vi "Complete Collection.vi"(8 "error in":errorcluster) -> (0 "error out":errorcluster)   [LabVIEW 2013]
uses:
  Collection Support/Controls/PED States.ctl
  Collection Support/Controls/FirstCall.ctl
panel:
  in  "Trial Duration (s)":dbl=10.0 format="%#_13g"
  in  "Exit Button":bool
  in  "Longest Time Between Interruptions":dbl=1.3 format="%#_13g"
  in  "Starting Second":dbl=3.4 format="%#_13g"
  in  "Interruptions":i32
  in  "Delay":u32
  in  "Shortest Time Between Interruptions":dbl=0.8 format="%#_13g"
  out "Countdown":dbl format="%#.0g"
  out "Audio Chart":dynamicdata(graph)
  out "Pressure Chart":dynamicdata(graph)
  in  "START/STOP":bool
  in  "Stopped?":bool
  out "STOP":bool
  out "GO":bool
  # "- You can set the delay and number of interruptions to 0 to test labial interruptions\n\n-The starting second sets how long after GO the first interruption will be\n\n-The longest time between interrruptions sets the maximum amount of time between interruptions\n\n-The shortest time between interruptions sets the minimum time between interruptions. If you want quicker intteruptions, lower this value."
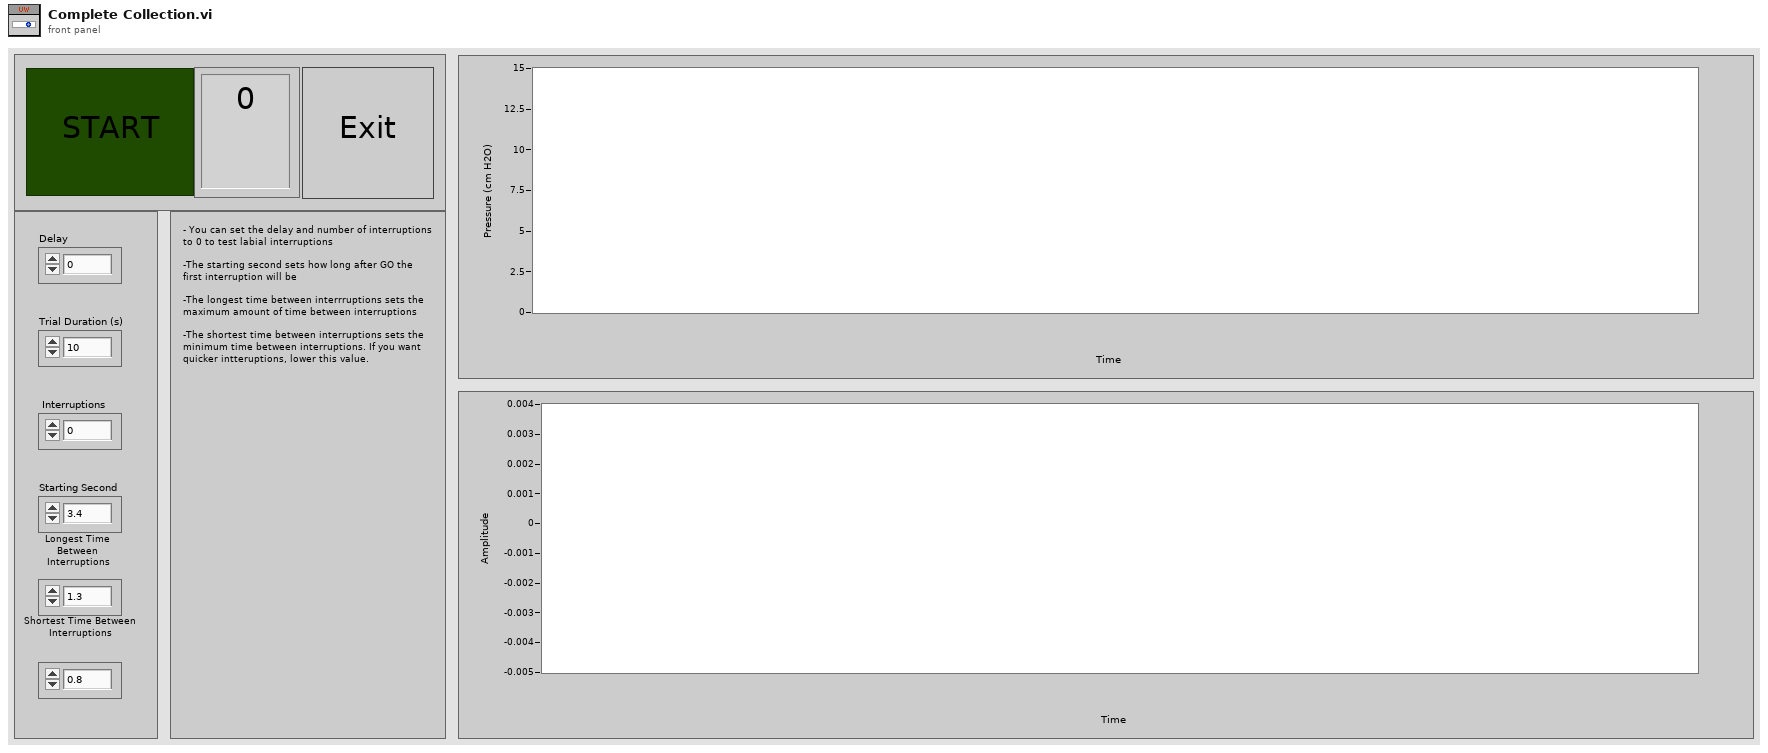
[diagram p1: front panel]
types:
  T1 = enum16{"open", "replace", "create", "open or create", "replace or create", "replace or create with confirmation"}
  T2 = typedef "PED States.ctl" = enum16{"Initialize", "Wait", "Record", "Save", "Reset", "Exit"}
  T3 = typedef "FirstCall.ctl" = enum16{"First", "After"}
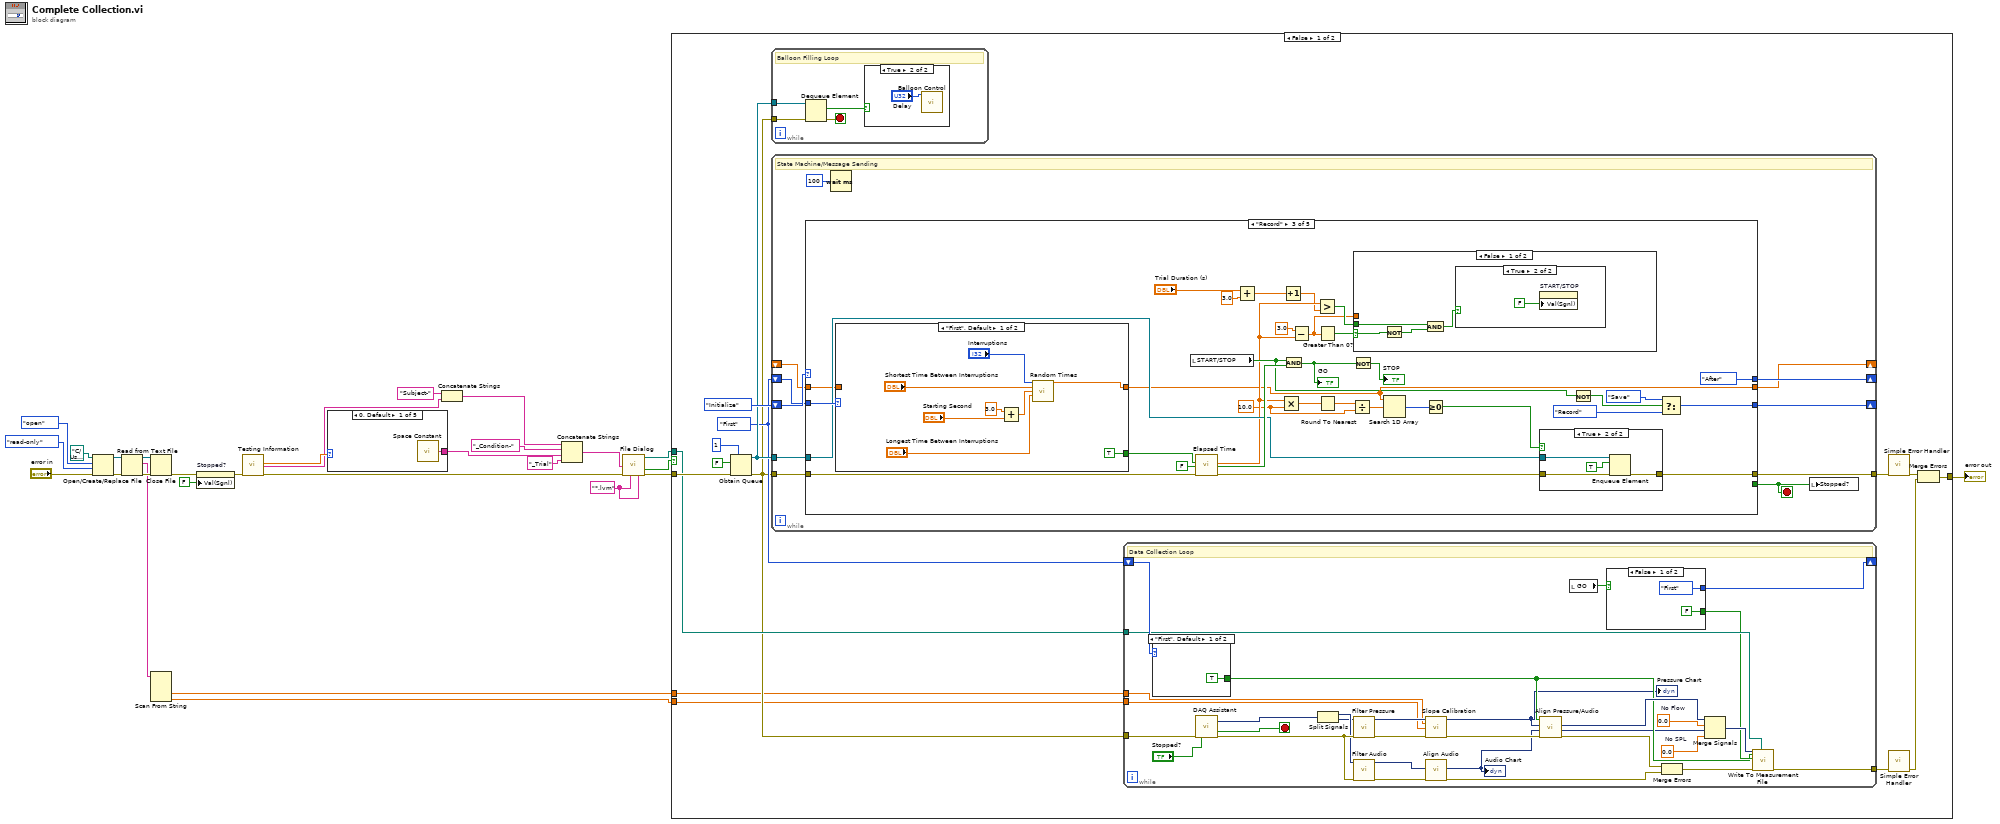
[diagram p0: block diagram]
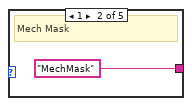
[diagram p2: hidden frame]
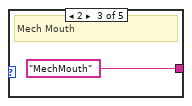
[diagram p3: hidden frame]
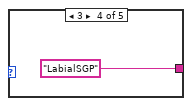
[diagram p4: hidden frame]
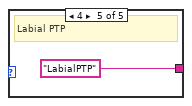
[diagram p5: hidden frame]
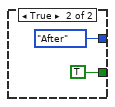
[diagram p6: hidden frame]
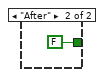
[diagram p7: hidden frame]
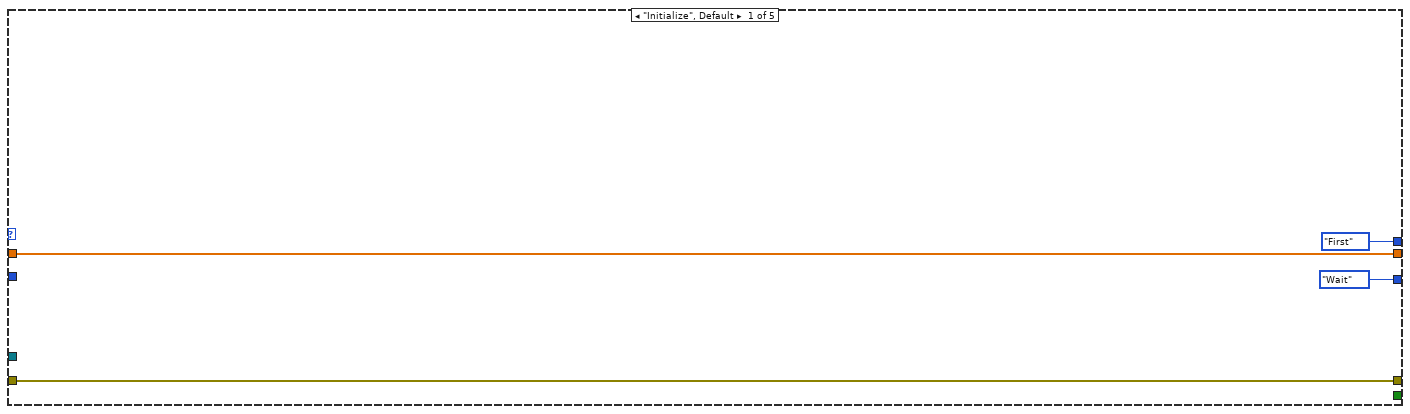
[diagram p9: hidden frame]
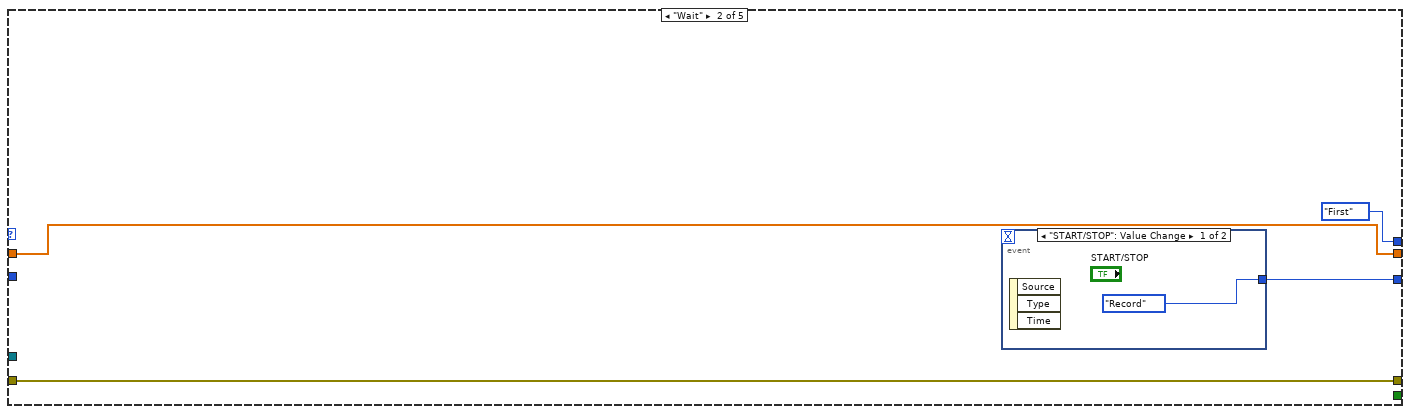
[diagram p10: hidden frame]
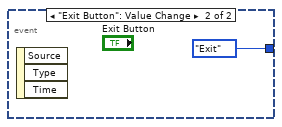
[diagram p11: hidden frame]
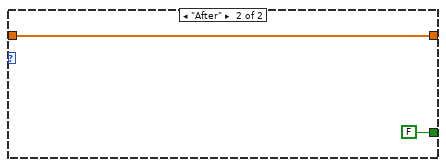
[diagram p13: hidden frame]
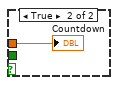
[diagram p15: hidden frame]
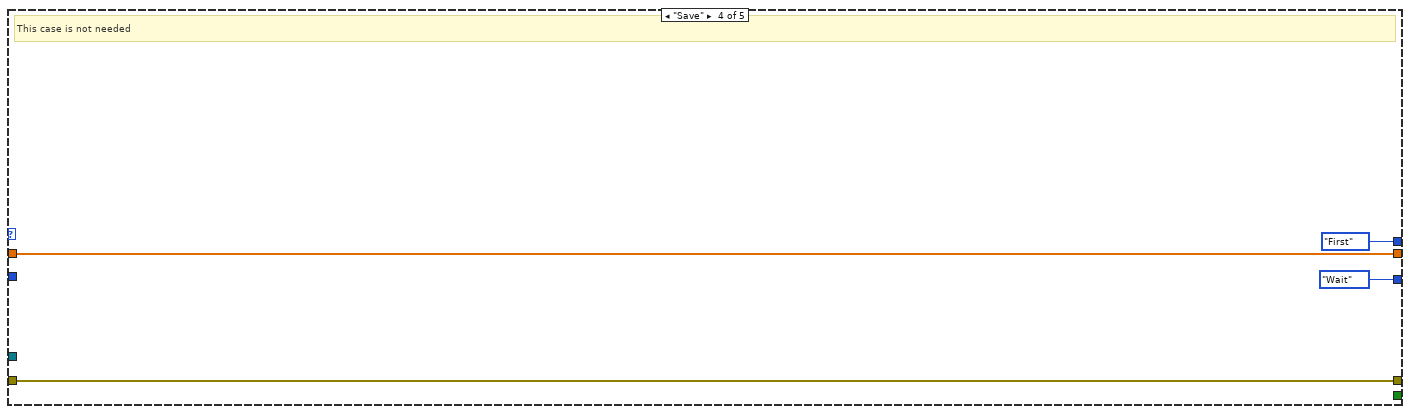
[diagram p16: hidden frame]
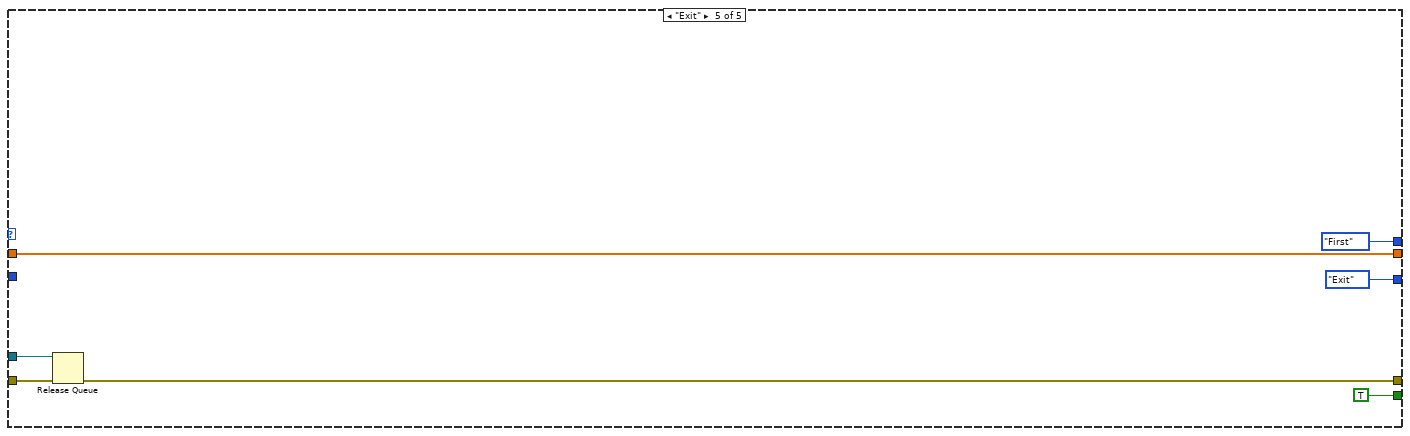
[diagram p17: hidden frame]
diagram:
  w26 = "*.lvm" ("pattern label")
  n1 = Open/Create/Replace File(file path (use dialog)=path "C:/Users/scholp/Desktop/Calibration .txt files/Calibration Values.txt", error in="error in", operation (0:open)=T1."open", access (0:read/write)=enum16{"read/write", "read-only", "write-only"}."read-only") -> (refnum out=w20:refnum<file>, error out=w24:errorcluster)  [unwired: 2 in, 1 out]
  n2 = Read from Text File(file (use dialog)=w20, error in=w24) -> (refnum out=w18:refnum<file>, text=w17:string, error out=w23:errorcluster)  [unwired: 2 in, 1 out]
  n3 = Close File(refnum=w18, error in=w23) -> (error out=w14:errorcluster)  [unwired: 1 out]
  n4 = Scan From String(input string=w17) -> (output 1=w16:dbl, output 2=w15:dbl)  [unwired: 5 in, 3 out]
  n5 = property on="Stopped?" class="Bool (strict)"(error in=w14, "Val(Sgnl)"=FALSE ("Value (Signaling)")) -> (error out=w1:errorcluster)  [unwired: 1 in, 1 out]
  n6 = call "Testing Information"("error in (no error)"=w1) -> ("Condition"=w10:dbl, "Subject"=w8:string, "error out"=w2:errorcluster)  [unwired: 15 in, 1 out]
  n7 = case shown="0, Default" w10 {
    tunnel: [w29 "MechMask" ("string") "MechMouth" ("string") "LabialSGP" ("string") "LabialPTP" ("string")] -> w7
    frame 0, Default {
      n8 = call <vilib>:"Space Constant.vi"() -> ("String"=w29:string)
    }
    frame 1 {
      # "Mech Mask"
    }
    frame 2 {
      # "Mech Mouth"
    }
    frame 3 {
    }
    frame 4 {
      # "Labial PTP"
    }
  }
  n9 = Concatenate Strings("Subject-" ("default name"), w8) -> (w4:string)
  n10 = Concatenate Strings(w4, "_Condition-" ("string"), w7, "_Trial" ("string")) -> (w3:string)
  n11 = call "File Dialog"("default name"=w3, "error in"=w2, "pattern (all files)"=w26, "pattern label"=w26) -> ("selected path"=w27:path, "cancelled"=w12:bool, "error out"=w28:errorcluster)  [unwired: 8 in, 1 out]
  n12 = case shown="False" w12 {
    tunnel: w28 -> [w43 w177]
    tunnel: w27 -> [w42 _]
    tunnel: w16 -> [w38 _]
    tunnel: w15 -> [w37 _]
    tunnel: [w34 w177] -> w11
    frame False {
      w44 = FirstCall."First"
      n13 = Obtain Queue(max queue size (-1, unlimited)=1, element data type=FALSE, error in (no error)=w43) -> (queue out=w45:refnum<queue>, error out=w41:errorcluster)  [unwired: 2 in, 1 out]
      n14 = while {
        tunnel: w45 -> [w87]
        tunnel: w41 -> [w86]
        stop <- w88 stop-if-true
        # "Balloon Filling Loop"
        n15 = Dequeue Element(queue=w87, error in (no error)=w86) -> (element=w89:bool, error out=w88:errorcluster)  [unwired: 1 in, 2 out]
        n16 = case shown="True" w89 {
          frame False {
          }
          frame True {
            n17 = call "Balloon Control.vi"("Delay (ms)"="Delay") -> ()  [unwired: 11 in]
          }
        }
      }
      n18 = while {
        shift-right: [w101] -> _
        shift-left: PED_States."Initialize" -> [w100]
        tunnel: w45 -> [w97]
        tunnel: w41 -> [w99]
        shift-right: [w96] -> _
        shift-left: w44 -> [w98]
        tunnel: [w94] -> w39
        shift-right: [w91] -> _
        shift-left: _ -> [w92]
        stop <- w95 stop-if-true
        # "State Machine/Message Sending"
        n19 = case shown="\"Record\"" w100 {
          tunnel: [_ _ _ _ TRUE] -> w95
          tunnel: [PED_States."Wait" ("f") w109 w128 PED_States."Wait" ("element") PED_States."Exit" ("element")] -> w101
          tunnel: w99 -> [w103 w106 w134 w167 w174]
          tunnel: w98 -> [_ _ w130 _ _]
          tunnel: w97 -> [_ _ w122 _ w173]
          tunnel: [FirstCall."First" FirstCall."First" FirstCall."After" FirstCall."First" FirstCall."First"] -> w96
          tunnel: [w102 w107 w118 w166 w170] -> w91
          tunnel: [w103 w106 w121 w167 w171] -> w94
          tunnel: w92 -> [w102 w107 w117 w166 w170]
          frame "Initialize", Default {
          }
          frame "Wait" {
            n20 = event shown="[0] \"START/STOP\": Value Change" {
              selector: _ -> [_ _]
              dyn-events: _ -> [_ _]
              timeout: _ -> [_ _]
              tunnel: [PED_States."Record" ("element") PED_States."Exit" ("element")] -> w109
              event "START/STOP": Value Change {
                n21 = event-data() -> ()  [unwired: 1 in, 3 out]
              }
              event "Exit Button": Value Change {
                n22 = event-data() -> ()  [unwired: 1 in, 3 out]
              }
            }
          }
          frame "Record" {
            w112 = 10.0 ("x")
            n23 = case shown="\"First\", Default" w130 {
              tunnel: [TRUE FALSE] -> w131
              tunnel: [w156 w158] -> w118
              tunnel: w117 -> [_ w158]
              frame "First", Default {
                n24 = Add(x=3.0, y="Starting Second") -> (x+y=w150:dbl)
                n25 = call "Random Times.vi"("Number of Interruptions"="Interruptions", "Start Second"="Shortest Time Between Interruptions", "Longest Gap"=w150, "Shortest Gap"="Longest Time Between Interruptions") -> ("Interruption TImes"=w156:dbl[])  [unwired: 10 in, 1 out]
              }
              frame "After" {
              }
            }
            n26 = local read "START/STOP"() -> (w135:bool)
            n27 = call "Elapsed Time"("Reset"=w131, "Auto Reset"=FALSE, "error in (no error)"=w134) -> ("Elapsed Time (s)"=w120:dbl, "Time has Elapsed"=w138:bool, "error out"=w123:errorcluster)  [unwired: 9 in, 5 out]
            n28 = Add(x="Trial Duration (s)", y=3.0) -> (x+y=w113:dbl)
            n29 = Multiply(x=w120, y=w112) -> (x*y=w125:dbl)
            n30 = Increment(x=w113) -> (x+1=w116:dbl)
            n31 = And(x=w135, y=w138) -> (x .and. y?=w137:bool)
            "GO" <- w137
            n32 = Subtract(x=3.0, y=w120) -> (x-y=w139:dbl)
            n33 = Greater?(x=w120, y=w116) -> (0:w141:bool)
            n34 = Greater Than 0?(x=w139) -> (x > 0?=w142:bool)
            n35 = Round To Nearest(number=w125) -> (nearest integer value=w124:dbl)
            n36 = Divide(x=w124, y=w112) -> (x/y=w126:dbl)
            n37 = Not(x=w137) -> (.not. x?=→"STOP":bool)
            n38 = case shown="False" w142 {
              selector: w142 -> [w161 _]
              tunnel: w139 -> [_ w165]
              tunnel: w141 -> [w163 _]
              frame False {
                n39 = Not(x=w161) -> (.not. x?=w160:bool)
                n40 = And(x=w163, y=w160) -> (x .and. y?=w162:bool)
                n41 = case shown="True" w162 {
                  frame False {
                  }
                  frame True {
                    n42 = property on="START/STOP" class="Bool (strict)"("Val(Sgnl)"=FALSE ("Value (Signaling)")) -> ()  [unwired: 2 in, 2 out]
                  }
                }
              }
              frame True {
                "Countdown" <- w165
              }
            }
            n43 = Search 1D Array(1D array=w118, element=w126) -> (index of element=w127:i32)  [unwired: 1 in]
            n44 = Greater Or Equal To 0?(x=w127) -> (x >= 0?=w119:bool)
            n45 = case shown="True" w119 {
              tunnel: [w145 w149] -> w121
              tunnel: w123 -> [w145 w148]
              tunnel: w122 -> [_ w147]
              frame False {
              }
              frame True {
                n46 = Enqueue Element(queue=w147, element=TRUE, error in (no error)=w148) -> (error out=w149:errorcluster)  [unwired: 1 in, 2 out]
              }
            }
            n47 = Not(x=w135) -> (.not. x?=w133:bool)
            n48 = Select(t=PED_States."Save" ("f"), s=w133, f=PED_States."Record") -> (s? t:f=w128:T2)
          }
          frame "Save" {
            # "This case is not needed"
          }
          frame "Exit" {
            n49 = Release Queue(queue=w173, error in (no error)=w174) -> (error out=w171:errorcluster)  [unwired: 1 in, 2 out]
          }
        }
        n50 = Wait (ms)(milliseconds to wait=u32 100) -> ()  [unwired: 1 out]
        n51 = local write "Stopped?"(w95) -> ()
      }
      n52 = while {
        tunnel: w41 -> [w72]
        shift-right: [w66] -> _
        shift-left: w44 -> [w68]
        tunnel: w42 -> [w65]
        tunnel: [w61] -> w40
        tunnel: w38 -> [w60]
        tunnel: w37 -> [w59]
        stop <- w73 stop-if-true
        w55 = 0.0  # No SPL
        w56 = 0.0  # No Flow
        # "Data Collection Loop"
        n53 = case shown="\"First\", Default" w68 {
          tunnel: [TRUE FALSE] -> w52
          frame "First", Default {
          }
          frame "After" {
          }
        }
        n54 = call "DAQ Assistant"("error in"=w72, "stop (F)"="Stopped?") -> ("data"=w76:dynamicdata, "stopped"=w73:bool, "error out"=w58:errorcluster)  [unwired: 14 in, 1 out]
        n55 = Split Signals(w76) -> (w54:dynamicdata, w53:dynamicdata)  [unwired: 2 in]
        n56 = call "Filter Pressure"("error in (no error)"=w58, "Signal"=w53) -> ("error out"=w75:errorcluster, "Filtered Signal"=w79:dynamicdata)  [unwired: 8 in]
        n57 = call "Filter Audio"("error in (no error)"=w58, "Signal"=w54) -> ("error out"=w77:errorcluster, "Filtered Signal"=w78:dynamicdata)  [unwired: 8 in]
        n58 = call "Slope Calibration.vi"("Voltage"=w79, "Slope"=w60, "Intercept"=w59, "error in (no error)"=w75) -> ("Result"=w49:dynamicdata, "error out"=w74:errorcluster)  [unwired: 10 in]
        "Pressure Chart" <- w49
        n59 = call "Align Audio"("error in (no error)"=w77, "Signals"=w78) -> ("error out"=w69:errorcluster, "Resampled Signals"=w51:dynamicdata)  [unwired: 7 in, 1 out]
        "Audio Chart" <- w51
        n60 = call "Align Pressure/Audio"("error in (no error)"=w74, "Signals 2"=w51, "Signals"=w49, "Reset"=w52) -> ("error out"=w70:errorcluster, "Resampled Signals 2"=w50:dynamicdata, "Resampled Signals"=w57:dynamicdata)  [unwired: 5 in]
        n61 = local read "GO"() -> (w67:bool)
        n62 = case shown="False" w67 {
          tunnel: [FirstCall."First" FirstCall."After"] -> w66
          tunnel: [FALSE TRUE] -> w62
          frame False {
          }
          frame True {
          }
        }
        n63 = Merge Errors(w70, w69) -> (w63:errorcluster)
        n64 = Merge Signals(w57, w56, w50, w55) -> (w64:dynamicdata)
        n65 = call "Write To Measurement File"("Signals"=w64, "Reset"=w52, "Enable"=w62, "error in (no error)"=w63, "Filename"=w65) -> ("error out"=w61:errorcluster)  [unwired: 12 in, 2 out]
      }
      n66 = call <vilib>:"Simple Error Handler.vi"("error in (no error)"=w39) -> ("error out"=w36:errorcluster)  [unwired: 4 in, 4 out]
      n67 = call <vilib>:"Simple Error Handler.vi"("error in (no error)"=w40) -> ("error out"=w35:errorcluster)  [unwired: 4 in, 4 out]
      n68 = Merge Errors(w36, w35) -> (w34:errorcluster)
    }
    frame True {
    }
  }
  "error out" <- w11
